vi "Remove SLSC Module.vi"(8 "error in (no error)":errorcluster, 11 "SLSC Module":u64) -> (0 "error out":errorcluster, 3 "SLSC Module out":u64)   [LabVIEW 2017, in "VeriStand SLSC Scripting.lvlib"]
uses:
  VeriStand SLSC Scripting.lvlib
  NationalInstruments.VeriStand.SystemDefinitionAPI
  NationalInstruments.VeriStand.SystemStorage
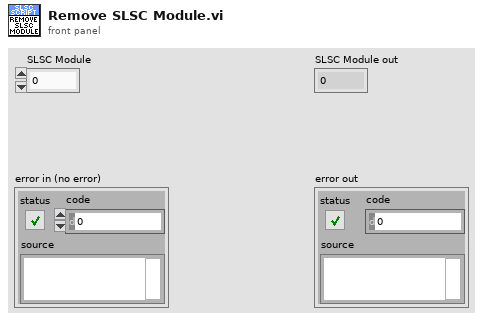
[diagram p1: front panel]
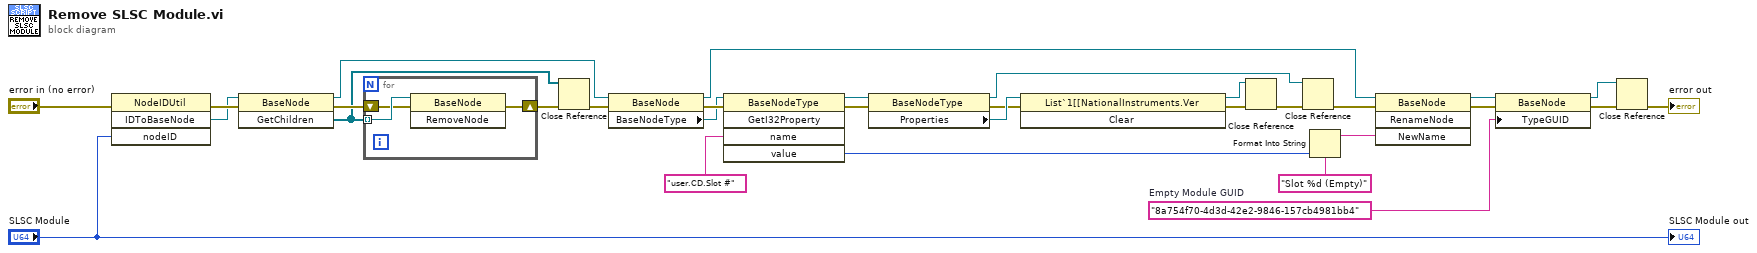
[diagram p0: block diagram]
diagram:
  w2 = "8a754f70-4d3d-42e2-9846-157cb4981bb4"  # Empty Module GUID
  n1 = invoke class="NodeIDUtil" method="IDToBaseNode"(error in="error in (no error)", "nodeID"="SLSC Module") -> (error out=w29:errorcluster, "IDToBaseNode"=w28:refnum<k24>)  [unwired: 2 in, 2 out]
  n2 = invoke class="BaseNode" method="GetChildren"(reference=w28, error in=w29) -> (reference out=w25:refnum<k24>, error out=w27:errorcluster, "GetChildren"=w21:refnum<k24>[])  [unwired: 1 in]
  n3 = for {
    tunnel: w21 -> [w34] mode=indexing
    shift-right: [w32] -> w26
    shift-left: w27 -> [w33]
    n4 = invoke class="BaseNode" method="RemoveNode"(reference=w34, error in=w33) -> (error out=w32:errorcluster)  [unwired: 1 in, 2 out]
  }
  n5 = Close Reference(reference=w21, error in (no error)=w26) -> (error out=w22:errorcluster)
  n6 = property class="BaseNode"(reference=w25, error in=w22) -> (reference out=w15:refnum<k24>, error out=w10:errorcluster, "BaseNodeType"=w7:refnum<k24>)
  n7 = invoke class="BaseNodeType" method="GetI32Property"(reference=w7, error in=w10, "name"="user.CD.Slot #") -> (reference out=w9:refnum<k24>, error out=w8:errorcluster, "value"=w6:i32)  [unwired: 2 in, 2 out]
  n8 = property class="BaseNodeType"(reference=w9, error in=w8) -> (reference out=w17:refnum<k24>, error out=w20:errorcluster, "Properties"=w24:refnum<k24>)
  n9 = invoke class="List`1[[NationalInstruments.Ver" method="Clear"(reference=w24, error in=w20) -> (reference out=w19:refnum<k24>, error out=w23:errorcluster)  [unwired: 1 in, 1 out]
  n10 = Close Reference(reference=w19, error in (no error)=w23) -> (error out=w18:errorcluster)
  n11 = Close Reference(reference=w17, error in (no error)=w18) -> (error out=w16:errorcluster)
  n12 = Format Into String(format string="Slot %d (Empty)", w6) -> (resulting string=w12:string)  [unwired: 2 in, 1 out]
  n13 = invoke class="BaseNode" method="RenameNode"(reference=w15, error in=w16, "NewName"=w12) -> (reference out=w3:refnum<k24>, error out=w5:errorcluster)  [unwired: 1 in, 2 out]
  n14 = property class="BaseNode"(reference=w3, error in=w5, "TypeGUID"=w2) -> (reference out=w1:refnum<k24>, error out=w4:errorcluster)
  n15 = Close Reference(reference=w1, error in (no error)=w4) -> (error out=→"error out":errorcluster)
  "SLSC Module out" <- "SLSC Module"
